vi "Save-Load Initial MovCor Values.vi"(6 "Which file? (User profile.ini)":T1=enum."Loaded User profile.ini", 8 "error in":errorcluster, 11 "Function":T2=enum."Load from file") -> (0 "error out":errorcluster)   [LabVIEW 2020]
uses:
  Typedefs/Save-Load enum.ctl
  Typedefs/Which path.ctl
  <vilib>/Utility/config.llb/NI_LVConfig.lvlib
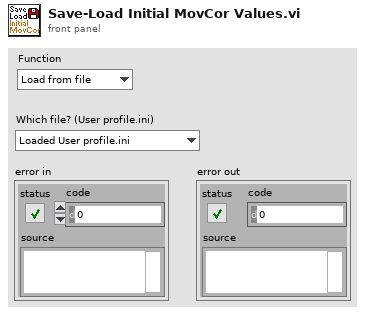
[diagram p1: front panel]
types:
  T1 = typedef "Which path.ctl" = enum16{"Configuration Files", "Calibration Files", "Images", "Setup.ini", "Loaded User profile.ini", "User's-Previous session.ini", "New user profile.ini", "Selected User profile.ini", "User profiles folder", "Power meter scaling.txt", "FOV Cal.ini", "Calibration.ini"}
  T2 = typedef "Save-Load enum.ctl" = enum16{"Save to file", "Load from file", "Compare from file", "Save Backup"}
  T3 = typedef "Ini file interface (DBL).ctl" = cluster{"key":string, "Save?":bool, "Default":dbl}[]
  T4 = typedef "Ini file interface (String).ctl" = cluster{"key":string, "Save?":bool, "Default":string}[]
  T5 = typedef "Ini file interface (Boolean).ctl" = cluster{"key":string, "Save?":bool, "Default":bool}[]
  T6 = typedef "NI_LVConfig.lvlib/Config Data RefNum.ctl" = refnum<k1>
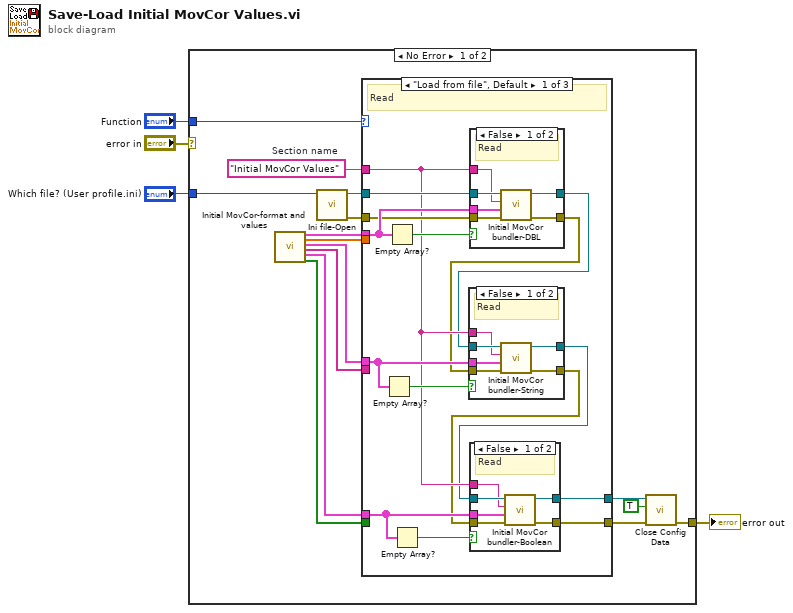
[diagram p0: block diagram]
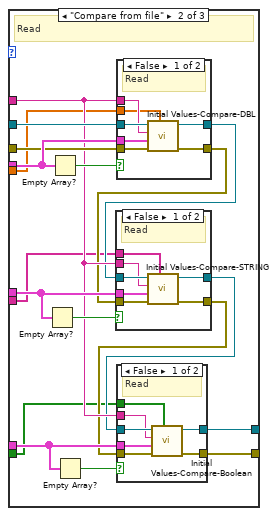
[diagram p5: hidden frame]
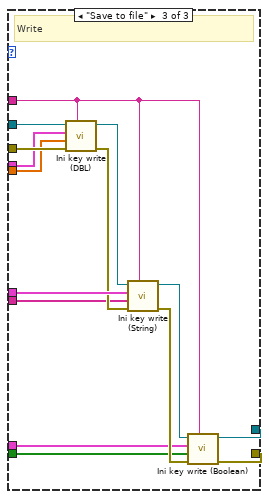
[diagram p9: hidden frame]
diagram:
  n1 = case shown="No Error" "error in" {
    selector: "error in" -> [_ w119]
    tunnel: [w13 w119] -> w4
    tunnel: "Function" -> [w6 _]
    tunnel: "Which file? (User profile.ini)" -> [w5 _]
    frame No Error {
      w19 = "Initial MovCor Values"  # Section name
      n2 = call "Initial MovCor-format and values.vi"() -> ("Ini file interface (DBL)"=w12:T3, "DBL values"=w11:dbl[], "String"=w10:T4, "String values"=w9:string[], "Boolean"=w8:T5, "Boolean values"=w7:bool[])  [unwired: 14 in]
      n3 = call "Ini file-Open.vi"("Which file?"=w5) -> ("error out"=w16:errorcluster, "User profile ini file ref"=w17:T6)  [unwired: 7 in, 2 out]
      n4 = case shown="\"Load from file\", Default" w6 {
        tunnel: [w29 w71 w105] -> w14
        tunnel: [w30 w72 w104] -> w15
        tunnel: w16 -> [w31 w73 w117]
        tunnel: w17 -> [w34 w76 w118]
        tunnel: w19 -> [w24 w66 w107]
        tunnel: w12 -> [w33 w75 w115]
        tunnel: w11 -> [_ w59 w116]
        tunnel: w7 -> [_ w61 w106]
        tunnel: w8 -> [w28 w70 w108]
        tunnel: w9 -> [_ w60 w111]
        tunnel: w10 -> [w25 w67 w114]
        frame "Load from file", Default {
          # "Read"
          n5 = Empty Array?(array=w25) -> (empty?=w26:bool)
          n6 = Empty Array?(array=w33) -> (empty?=w32:bool)
          n7 = Empty Array?(array=w28) -> (empty?=w27:bool)
          n8 = case shown="False" w32 {
            tunnel: w34 -> [w56 w58]
            tunnel: [w55 w58] -> w20
            tunnel: [w54 w57] -> w21
            tunnel: w31 -> [w53 w57]
            tunnel: w24 -> [w51 _]
            tunnel: w33 -> [w52 _]
            frame False {
              # "Read"
              n9 = call "Initial MovCor bundler-DBL.vi"("error in (no error)"=w53, "Ini file interface"=w52, "Section name"=w51, "Setup.ini ref"=w56) -> ("error out"=w54:errorcluster, "Setup.ini ref"=w55:T6)  [unwired: 6 in]
            }
            frame True {
              # "No parametersof such type"
            }
          }
          n10 = case shown="False" w26 {
            tunnel: [w37 w42] -> w23
            tunnel: [w36 w41] -> w22
            tunnel: w25 -> [w39 _]
            tunnel: w20 -> [w40 w42]
            tunnel: w21 -> [w35 w41]
            tunnel: w24 -> [w38 _]
            frame False {
              # "Read"
              n11 = call "Initial MovCor bundler-String.vi"("error in (no error)"=w35, "String"=w39, "Section name"=w38, "Refnum in"=w40) -> ("error out"=w36:errorcluster, "Refnum out"=w37:T6)  [unwired: 6 in]
            }
            frame True {
              # "No parametersof such type"
            }
          }
          n12 = case shown="False" w27 {
            tunnel: [w47 w50] -> w30
            tunnel: [w46 w49] -> w29
            tunnel: w28 -> [w43 _]
            tunnel: w23 -> [w48 w50]
            tunnel: w22 -> [w45 w49]
            tunnel: w24 -> [w44 _]
            frame False {
              # "Read"
              n13 = call "Initial MovCor bundler-Boolean.vi"("error in (no error)"=w45, "Boolean"=w43, "Section name"=w44, "Refnum in"=w48) -> ("error out"=w46:errorcluster, "Refnum out"=w47:T6)  [unwired: 6 in]
            }
            frame True {
              # "No parametersof such type"
            }
          }
        }
        frame "Compare from file" {
          # "Read"
          n14 = Empty Array?(array=w67) -> (empty?=w68:bool)
          n15 = Empty Array?(array=w75) -> (empty?=w74:bool)
          n16 = Empty Array?(array=w70) -> (empty?=w69:bool)
          n17 = case shown="False" w74 {
            tunnel: w76 -> [w101 w103]
            tunnel: [w100 w103] -> w62
            tunnel: [w99 w102] -> w63
            tunnel: w73 -> [w98 w102]
            tunnel: w66 -> [w96 _]
            tunnel: w75 -> [w97 _]
            tunnel: w59 -> [w95 _]
            frame False {
              # "Read"
              n18 = call "Initial Values-Compare-DBL.vi"("Current values"=w95, "error in (no error)"=w98, "Keys Array"=w97, "Section name"=w96, "User profile ini file ref"=w101) -> ("error out"=w99:errorcluster, "User profile ini file ref"=w100:T6)  [unwired: 2 in, 3 out]
            }
            frame True {
              # "No parametersof such type"
            }
          }
          n19 = case shown="False" w68 {
            tunnel: [w80 w85] -> w65
            tunnel: [w79 w84] -> w64
            tunnel: w67 -> [w82 _]
            tunnel: w62 -> [w83 w85]
            tunnel: w63 -> [w78 w84]
            tunnel: w66 -> [w81 _]
            tunnel: w60 -> [w77 _]
            frame False {
              # "Read"
              n20 = call "Initial Values-Compare-STRING.vi"("Current values"=w77, "error in (no error)"=w78, "Keys Array"=w82, "Section name"=w81, "User profile ini file ref"=w83) -> ("error out"=w79:errorcluster, "User profile ini file ref"=w80:T6)  [unwired: 2 in, 3 out]
            }
            frame True {
              # "No parametersof such type"
            }
          }
          n21 = case shown="False" w69 {
            tunnel: [w91 w94] -> w72
            tunnel: [w90 w93] -> w71
            tunnel: w70 -> [w87 _]
            tunnel: w65 -> [w92 w94]
            tunnel: w64 -> [w89 w93]
            tunnel: w66 -> [w88 _]
            tunnel: w61 -> [w86 _]
            frame False {
              # "Read"
              n22 = call "Initial Values-Compare-Boolean.vi"("Current values"=w86, "error in (no error)"=w89, "Keys Array"=w87, "Section name"=w88, "User profile ini file ref"=w92) -> ("error out"=w90:errorcluster, "User profile ini file ref"=w91:T6)  [unwired: 2 in, 3 out]
            }
            frame True {
              # "No parametersof such type"
            }
          }
        }
        frame "Save to file" {
          # "Write"
          n23 = call "Ini key write (DBL).vi"("Section"=w107, "error in (no error)"=w117, "Values (DBL)"=w116, "Ini file interface"=w115, "Ini file refnum in"=w118) -> ("error out"=w112:errorcluster, "Ini file refnum out"=w113:T6)  [unwired: 5 in]
          n24 = call "Ini key write (String).vi"("Section"=w107, "error in (no error)"=w112, "Values (String)"=w111, "Ini file interface"=w114, "Ini file refnum in"=w113) -> ("error out"=w109:errorcluster, "Ini file refnum out"=w110:T6)  [unwired: 5 in]
          n25 = call "Ini key write (Boolean).vi"("Section"=w107, "error in (no error)"=w109, "Values (Boolean)"=w106, "Ini file interface"=w108, "Ini file refnum in"=w110) -> ("error out"=w105:errorcluster, "Ini file refnum out"=w104:T6)  [unwired: 5 in]
        }
      }
      n26 = call <vilib>:"Close Config Data.vi"("error in (no error)"=w14, "write file if changed (T)"=TRUE ("write configuration file? (F)"), "refnum"=w15) -> ("error out"=w13:errorcluster)  [unwired: 7 in, 1 out]
    }
    frame Error {
    }
  }
  "error out" <- w4
